vi "SetVoltage.vi"(3 "Voltage":dbl format="%.3f", 4 "error in":errorcluster, 5 "connection ID":refnum<k5>) -> (0 "False":bool, 1 "error out":errorcluster, 2 "connection ID out":refnum<k5>)   [LabVIEW 2013]
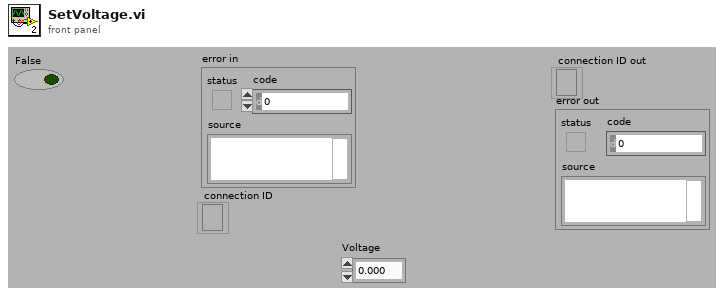
[diagram p1: front panel]
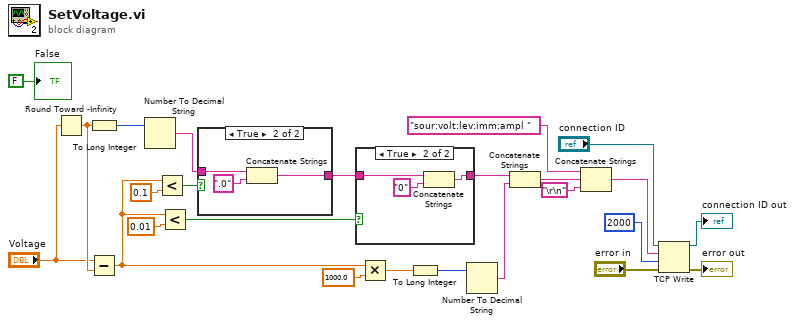
[diagram p0: block diagram]
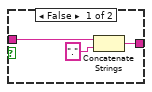
[diagram p3: hidden frame]
diagram:
  n1 = Round Toward -Infinity(1:"Voltage") -> (0:w16:dbl)
  n2 = To Long Integer(number=w16) -> (32bit integer=w14:i32)
  n3 = Subtract(x="Voltage", y=w16) -> (x-y=w9:dbl)
  n4 = Number To Decimal String(number=w14) -> (decimal integer string=w7:string)  [unwired: 1 out]
  n5 = Less?(x=w9, y=0.1) -> (x < y?=w8:bool)
  n6 = Less?(x=w9, y=0.01) -> (x < y?=w6:bool)
  n7 = case shown="True" w8 {
    tunnel: w7 -> [w27 w30]
    tunnel: [w26 w29] -> w5
    frame False {
      n8 = Concatenate Strings(w27, "." ("string")) -> (w26:string)
    }
    frame True {
      n9 = Concatenate Strings(w30, ".0" ("string")) -> (w29:string)
    }
  }
  n10 = case shown="True" w6 {
    tunnel: w5 -> [w32 w34]
    tunnel: [w32 w33] -> w4
    frame False {
    }
    frame True {
      n11 = Concatenate Strings(w34, "0" ("string")) -> (w33:string)
    }
  }
  n12 = Multiply(x=w9, y=1000.0) -> (x*y=w17:dbl)
  n13 = To Long Integer(number=w17) -> (32bit integer=w15:i32)
  n14 = Number To Decimal String(number=w15) -> (decimal integer string=w13:string)  [unwired: 1 out]
  n15 = Concatenate Strings(w4, w13) -> (w3:string)
  n16 = Concatenate Strings("sour:volt:lev:imm:ampl " ("data in"), w3, "\r\n") -> (w23:string)
  n17 = TCP Write(connection ID="connection ID", data in=w23, error in (no error)="error in", 9:2000 ("timeout ms (25000)")) -> (connection ID out=→"connection ID out":refnum<k5>, error out=→"error out":errorcluster)  [unwired: 1 out]
  "False" <- FALSE
